vi "CMD_APPLYSTAMP.vi"(6 "Gantry in":refnum<class "Gantry.lvclass">, 8 "error in (no error)":errorcluster, 10 "array":string[](array[string]), 11 "gScript Interpreter in":refnum<class "gScript Interpreter.lvclass">) -> (0 "error out":errorcluster, 3 "gScript Interpreter out":refnum<class "gScript Interpreter.lvclass">, 4 "Gantry out":refnum<class "Gantry.lvclass">)   [LabVIEW 2017, in "gScript Interpreter.lvclass"]
uses:
  gScript Interpreter.lvclass
  Shared Components/Gantry Class/Gantry.lvclass
  Shared Components/FlexWorktable/FlexWorktable.lvclass
  Shared Components/Vec3d Class/Vec3d.lvclass
  Shared Components/Orient3d Class/Orient3d.lvclass
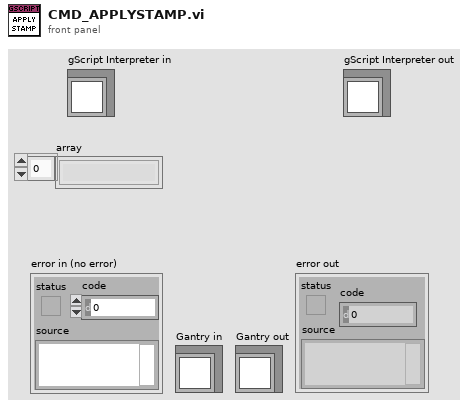
[diagram p1: front panel]
types:
  T1 = typedef "Memory Cell.ctl" = cluster{"type":T2, "x":dbl, "y":dbl, "z":dbl, "w":dbl}
  T2 = typedef "Memory Cell Type Enum.ctl" = enum16{"integer", "float", "vector", "rotation"}
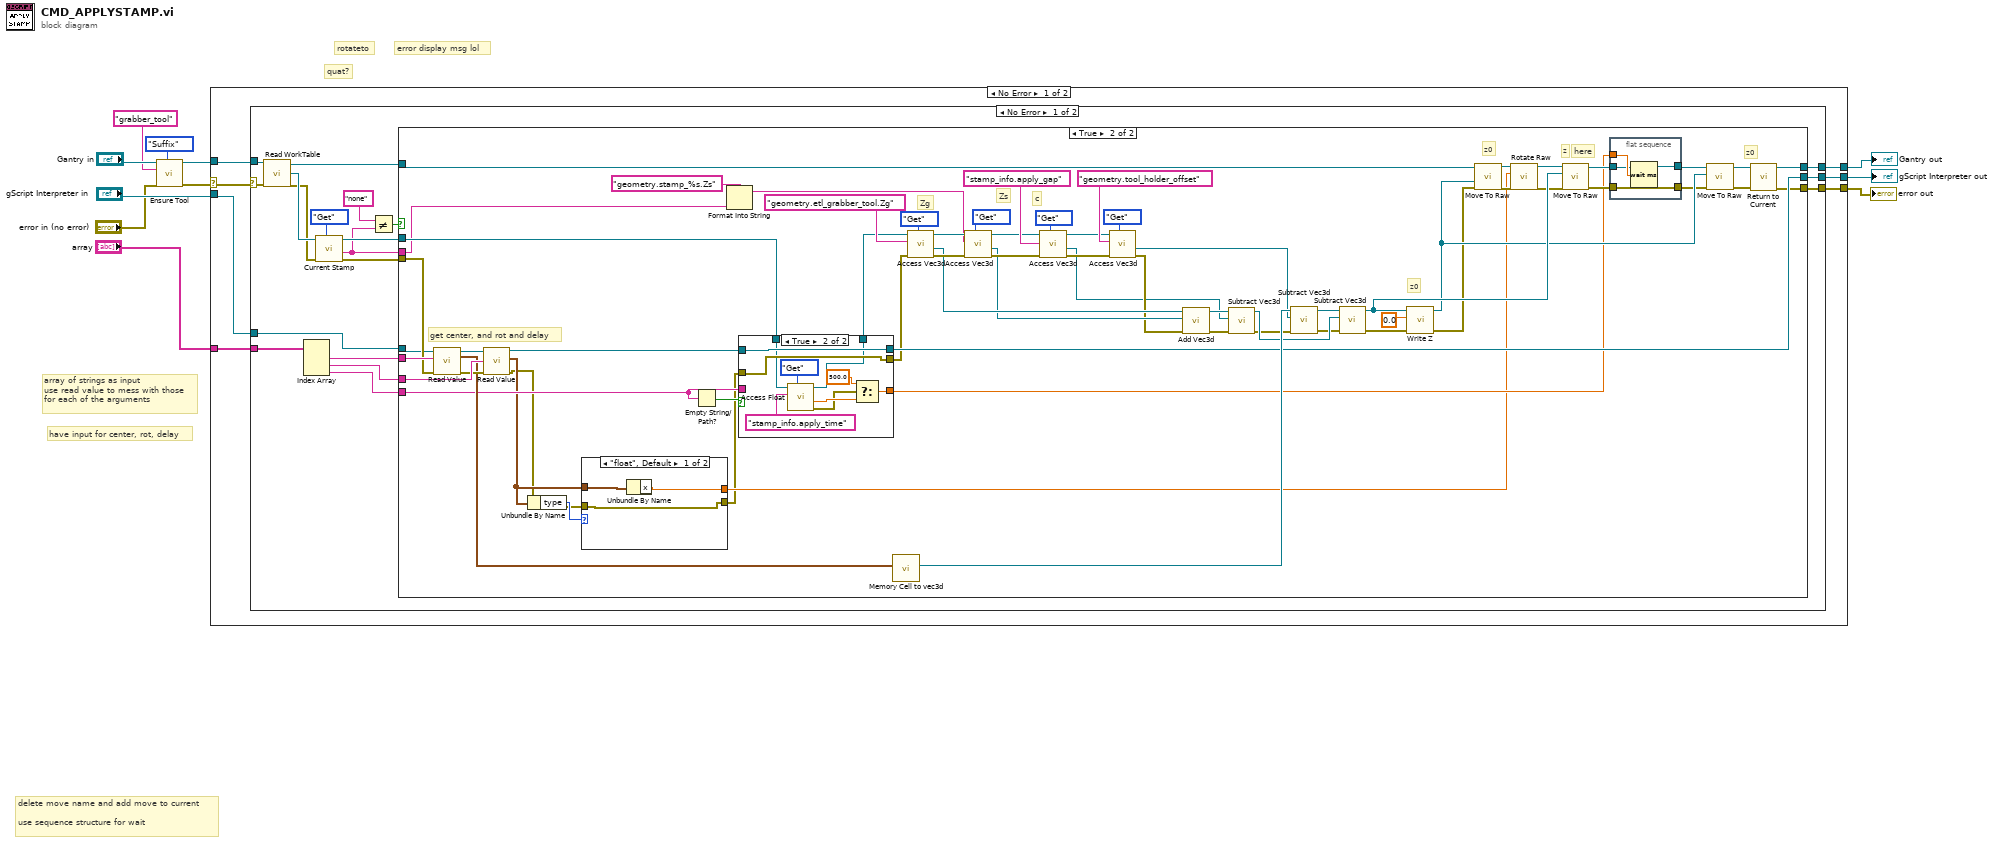
[diagram p0: block diagram]
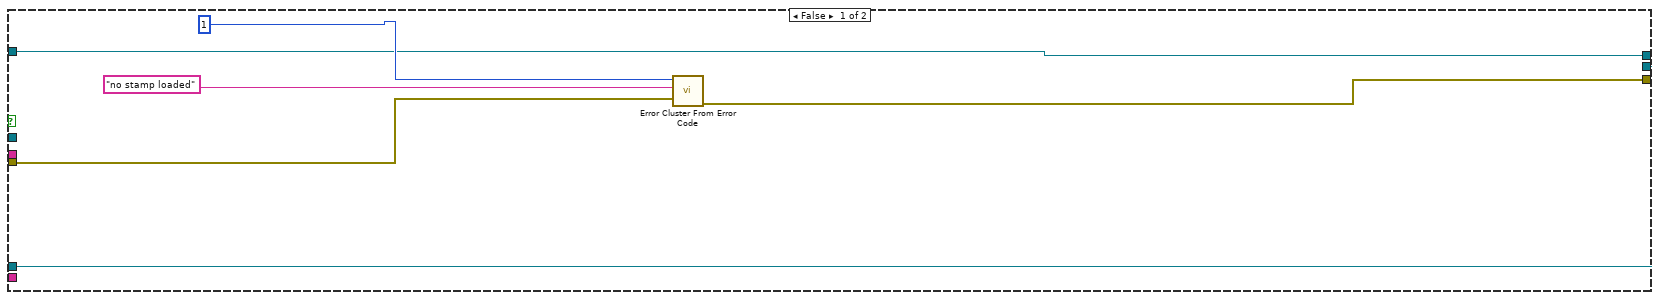
[diagram p2: hidden frame]
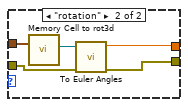
[diagram p3: hidden frame]
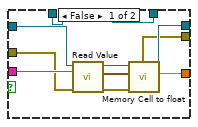
[diagram p4: hidden frame]
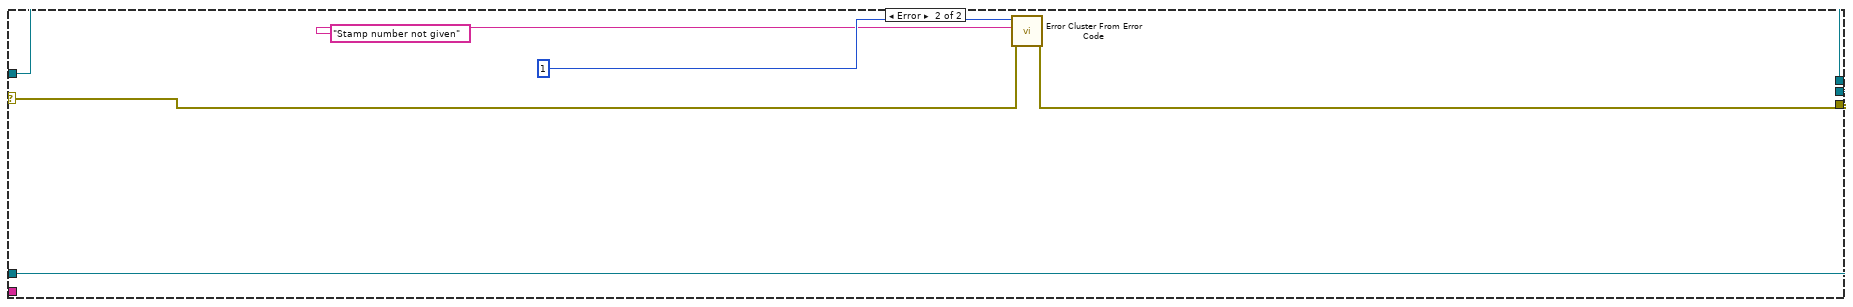
[diagram p5: hidden frame]
diagram:
  # "rotateto"
  # "quat?"
  # "error display msg lol"
  # "delete move name and add move to current\n\nuse sequence structure for wait"
  # "array of strings as input \nuse read value to mess with those\nfor each of the arguments"
  # "have input for center, rot, delay"
  n1 = call "Ensure Tool.vi"("Match Type"=enum16{"Full", "Suffix"}."Suffix", "error in (no error)"="error in (no error)", "Tool Name"="grabber_tool", "Gantry in"="Gantry in") -> ("error out"=w3:errorcluster, "Gantry out"=w6:refnum<class "Gantry.lvclass">)  [unwired: 6 in]
  n2 = case shown="No Error" w3 {
    selector: w3 -> [w16 w147]
    tunnel: [w18 w147] -> w11
    tunnel: [w12 w146] -> w9
    tunnel: "gScript Interpreter in" -> [w13 w146]
    tunnel: w6 -> [w15 w145]
    tunnel: [w17 w145] -> w8
    tunnel: "array" -> [w14 _]
    frame No Error {
      n3 = case shown="No Error" w16 {
        selector: w16 -> [w37 w141]
        tunnel: [w27 w142] -> w18
        tunnel: w15 -> [w36 w140]
        tunnel: [w28 w140] -> w17
        tunnel: w14 -> [w26 _]
        tunnel: w13 -> [w23 w139]
        tunnel: [w22 w139] -> w12
        frame No Error {
          n4 = call-dynamic "Read WorkTable.vi"("error in"=w37, "Gantry Class in"=w36) -> ("error out"=w31:errorcluster, "Worktable"=w35:refnum<class "FlexWorktable.lvclass">, "Gantry Class out"=w20:refnum<class "Gantry.lvclass">)  [unwired: 7 in]
          n5 = Index Array(array=w26) -> (element #1=w25:string, element #2=w24:string, element #3=w21:string)  [unwired: 3 in]
          n6 = call "Current Stamp.vi"("Get/Set"=enum16{"Get", "Set"}."Get", "error in (no error)"=w31, "FlexWorktable in"=w35) -> ("error out"=w33:errorcluster, "Current Stamp"=w19:string, "FlexWorktable out"=w32:refnum<class "FlexWorktable.lvclass">)  [unwired: 6 in]
          n7 = Not Equal?(x="none", y=w19) -> (x != y?=w30:bool)
          n8 = case shown="True" w30 {
            tunnel: [w40 w57] -> w27
            tunnel: w33 -> [w41 w98]
            tunnel: w20 -> [w39 w61]
            tunnel: [w39 w59] -> w28
            tunnel: w32 -> [_ w56]
            tunnel: w25 -> [_ w100]
            tunnel: w24 -> [_ w99]
            tunnel: w21 -> [_ w70]
            tunnel: w23 -> [w38 w92]
            tunnel: [w38 w68] -> w22
            tunnel: w19 -> [_ w47]
            frame False {
              n9 = call <vilib>:"Error Cluster From Error Code.vi"("error in (no error)"=w41, "error message (\"\")"="no stamp loaded" ("error message (\"\")"), "error code (0)"=1) -> ("error out"=w40:errorcluster)  [unwired: 6 in]
            }
            frame True {
              # "z0"
              # "z"
              # "z0"
              # "here"
              # "z0"
              # "c"
              # "Zs"
              # "Zg"
              # "get center, and rot and delay"
              n10 = call-dynamic "Read Value.vi"("error in (no error)"=w98, "String in"=w100, "gScript Interpreter in"=w92) -> ("error out"=w97:errorcluster, "Memory Cell"=w90:T1, "gScript Interpreter out"=w91:refnum<class "gScript Interpreter.lvclass">)  [unwired: 6 in]
              n11 = call-dynamic "Read Value.vi"("error in (no error)"=w97, "String in"=w99, "gScript Interpreter in"=w91) -> ("error out"=w50:errorcluster, "Memory Cell"=w51:T1, "gScript Interpreter out"=w69:refnum<class "gScript Interpreter.lvclass">)  [unwired: 6 in]
              n12 = Unbundle By Name(w51) -> ("type"=w53:T2)
              n13 = case shown="\"float\", Default" w53 {
                tunnel: [w111 w116] -> w52
                tunnel: [w110 w115] -> w49
                tunnel: w51 -> [w112 w114]
                tunnel: w50 -> [w110 w113]
                frame "float", Default {
                  n14 = Unbundle By Name(w112) -> ("x"=w111:dbl)
                }
                frame "rotation" {
                  n15 = call "Memory Cell to rot3d.vi"("Memory Cell"=w114) -> ("Orient3d out"=w117:refnum<class "Orient3d.lvclass">)  [unwired: 10 in]
                  n16 = call "To Euler Angles.vi"("error in"=w113, "Orient3d in"=w117) -> ("error out"=w115:errorcluster, "psi/yaw"=w116:dbl)  [unwired: 6 in, 2 out]
                }
              }
              n17 = Empty String/Path?(string/path=w70) -> (empty?=w71:bool)
              n18 = Format Into String(format string="geometry.stamp_%s.Zs", w47) -> (resulting string=w46:string)  [unwired: 2 in, 1 out]
              n19 = case shown="True" w71 {
                tunnel: [w124 w131] -> w54
                tunnel: w70 -> [w123 _]
                tunnel: w69 -> [w122 w130]
                tunnel: w49 -> [w121 w128]
                tunnel: [w120 w130] -> w68
                tunnel: [w119 w128] -> w67
                tunnel: w56 -> [w118 w127]
                tunnel: [w118 w126] -> w55
                frame False {
                  n20 = call-dynamic "Read Value.vi"("error in (no error)"=w121, "String in"=w123, "gScript Interpreter in"=w122) -> ("error out"=w119:errorcluster, "Memory Cell"=w125:T1, "gScript Interpreter out"=w120:refnum<class "gScript Interpreter.lvclass">)  [unwired: 6 in]
                  n21 = call "Memory Cell to float.vi"("Memory Cell"=w125) -> ("float out"=w124:dbl)  [unwired: 10 in]
                }
                frame True {
                  n22 = call-dynamic "Access Float.vi"("Get/Set"=enum16{"Get", "Set"}."Get", "Key"="stamp_info.apply_time", "FlexWorktable in"=w127) -> ("error out"=w129:errorcluster, "Value out"=w133:dbl, "FlexWorktable out"=w126:refnum<class "FlexWorktable.lvclass">)  [unwired: 6 in]
                  n23 = Select(t=500.0, s=w129, f=w133) -> (s? t:f=w131:dbl)
                }
              }
              n24 = call "Memory Cell to vec3d.vi"("Memory Cell"=w90) -> ("Vec3d out"=w89:refnum<class "Vec3d.lvclass">)  [unwired: 10 in]
              n25 = call-dynamic "Access Vec3d.vi"("Get/Set"=enum16{"Get", "Set"}."Get", "error in (no error)"=w67, "Key"="geometry.etl_grabber_tool.Zg", "FlexWorktable in"=w55) -> ("error out"=w104:errorcluster, "Value out"=w88:refnum<class "Vec3d.lvclass">, "FlexWorktable out"=w102:refnum<class "FlexWorktable.lvclass">)  [unwired: 5 in]
              n26 = call-dynamic "Access Vec3d.vi"("Get/Set"=enum16{"Get", "Set"}."Get", "error in (no error)"=w104, "Key"=w46, "FlexWorktable in"=w102) -> ("error out"=w103:errorcluster, "Value out"=w87:refnum<class "Vec3d.lvclass">, "FlexWorktable out"=w101:refnum<class "FlexWorktable.lvclass">)  [unwired: 5 in]
              n27 = call-dynamic "Access Vec3d.vi"("Get/Set"=enum16{"Get", "Set"}."Get", "error in (no error)"=w103, "Key"="stamp_info.apply_gap", "FlexWorktable in"=w101) -> ("error out"=w94:errorcluster, "Value out"=w44:refnum<class "Vec3d.lvclass">, "FlexWorktable out"=w93:refnum<class "FlexWorktable.lvclass">)  [unwired: 5 in]
              n28 = call-dynamic "Access Vec3d.vi"("Get/Set"=enum16{"Get", "Set"}."Get", "error in (no error)"=w94, "Key"="geometry.tool_holder_offset", "FlexWorktable in"=w93) -> ("error out"=w45:errorcluster, "Value out"=w83:refnum<class "Vec3d.lvclass">)  [unwired: 5 in, 1 out]
              n29 = call-dynamic "Add Vec3d.vi"("error in (no error)"=w45, 10:"Vec3d Class in"=w87, 11:"Vec3d Class in"=w88) -> ("error out"=w82:errorcluster, "Vec3d Class out"=w86:refnum<class "Vec3d.lvclass">)  [unwired: 7 in]
              n30 = call "Subtract Vec3d.vi"("error in (no error)"=w82, "Vec3d in 2"=w44, "Vec3d in 1"=w86) -> ("error out"=w81:errorcluster, "Vec3d Class out"=w84:refnum<class "Vec3d.lvclass">)  [unwired: 7 in]
              n31 = call "Subtract Vec3d.vi"("error in (no error)"=w81, "Vec3d in 2"=w83, "Vec3d in 1"=w89) -> ("error out"=w80:errorcluster, "Vec3d Class out"=w85:refnum<class "Vec3d.lvclass">)  [unwired: 7 in]
              n32 = call "Subtract Vec3d.vi"("error in (no error)"=w80, "Vec3d in 2"=w84, "Vec3d in 1"=w85) -> ("error out"=w79:errorcluster, "Vec3d Class out"=w74:refnum<class "Vec3d.lvclass">)  [unwired: 7 in]
              n33 = call-dynamic "Write Z.vi"("error in (no error)"=w79, "Z"=0.0, "Vec3d Class in"=w74) -> ("error out"=w62:errorcluster, "Vec3d Class out"=w72:refnum<class "Vec3d.lvclass">)  [unwired: 7 in]
              n34 = call-dynamic "Move To Raw.vi"("error in"=w62, "Destination"=w72, "Gantry in"=w61) -> ("error out"=w77:errorcluster, "Gantry out"=w76:refnum<class "Gantry.lvclass">)  [unwired: 7 in]
              n35 = call-dynamic "Rotate Raw.vi"("error in"=w77, "position(deg)"=w52, "Gantry in"=w76) -> ("error out"=w73:errorcluster, "Gantry out"=w75:refnum<class "Gantry.lvclass">)  [unwired: 7 in]
              n36 = call-dynamic "Move To Raw.vi"("error in"=w73, "Destination"=w74, "Gantry in"=w75) -> ("error out"=w64:errorcluster, "Gantry out"=w66:refnum<class "Gantry.lvclass">)  [unwired: 7 in]
              n37 = flat-sequence {
                tunnel: w54 -> [w138]
                tunnel: [w137] -> w65
                tunnel: w66 -> [w137]
                tunnel: w64 -> [w136]
                tunnel: [w136] -> w63
                frame #0 {
                  n38 = Wait (ms)(milliseconds to wait=w138) -> ()  [unwired: 1 out]
                }
              }
              n39 = call-dynamic "Move To Raw.vi"("error in"=w63, "Destination"=w72, "Gantry in"=w65) -> ("error out"=w58:errorcluster, "Gantry out"=w60:refnum<class "Gantry.lvclass">)  [unwired: 7 in]
              n40 = call-dynamic "Return to Current.vi"("error in"=w58, "Gantry in"=w60) -> ("error out"=w57:errorcluster, "Gantry out"=w59:refnum<class "Gantry.lvclass">)  [unwired: 8 in]
            }
          }
        }
        frame Error {
          n41 = call <vilib>:"Error Cluster From Error Code.vi"("error in (no error)"=w141, "error message (\"\")"="Stamp number not given" ("error message (\"\")"), "error code (0)"=1) -> ("error out"=w142:errorcluster)  [unwired: 6 in]
        }
      }
    }
    frame Error {
    }
  }
  "error out" <- w11
  "gScript Interpreter out" <- w9
  "Gantry out" <- w8
